vi "lectura comas2.vi"() -> ()   [LabVIEW 2021]
uses:
  <vilib>/Instr/_visa.llb/VISA Configure Serial Port (Instr).vi
panel:
  in  "PARO":bool
  in  "stop":bool
  out "BUFFER":string
  out "HUMEDAD":dbl(slide) scale=0.0..100.0
  out "TEMPERATURA":dbl(slide) scale=0.0..100.0
  in  "VISA resource name":refnum<visa-resource-name>
  in  "START":bool
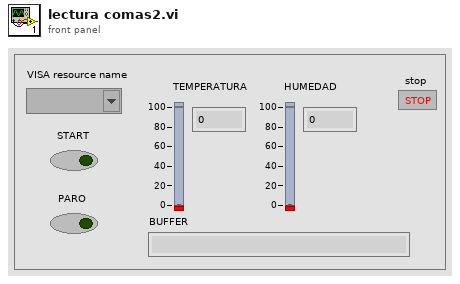
[diagram p1: front panel]
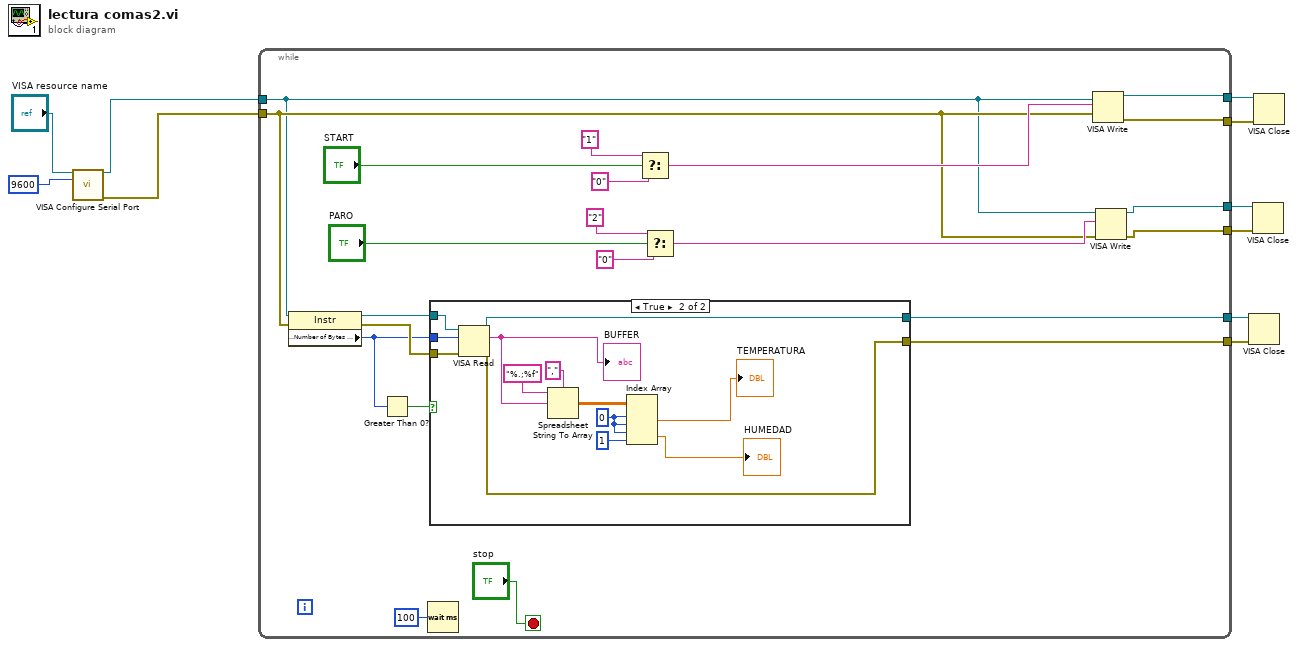
[diagram p0: block diagram]
diagram:
  n1 = call-poly "VISA Configure Serial Port"("VISA resource name"="VISA resource name", "baud rate (9600)"=u32 9600) -> ("VISA resource name out"=w10:refnum<visa-resource-name>, "error out"=w8:errorcluster)  [unwired: 12 in]
  n2 = while {
    tunnel: w10 -> [w13]
    tunnel: [w32] -> w9
    tunnel: w8 -> [w14]
    tunnel: [w31] -> w7
    tunnel: [w25] -> w4
    tunnel: [w24] -> w3
    tunnel: [w12] -> w2
    tunnel: [w11] -> w1
    stop <- "stop" stop-if-true
    n3 = property class="Instr"(reference=w13, error in=w14) -> (reference out=w21:refnum<visa-resource-name>, error out=w22:errorcluster, "Serial Settings:Number of Bytes at Serial Port"=w20:u32)
    n4 = Greater Than 0?(x=w20) -> (x > 0?=w19:bool)
    n5 = Wait (ms)(milliseconds to wait=u32 100) -> ()  [unwired: 1 out]
    n6 = case shown="True" w19 {
      tunnel: [w34 w39] -> w25
      tunnel: [w33 w38] -> w24
      tunnel: w22 -> [w33 w37]
      tunnel: w20 -> [_ w36]
      tunnel: w21 -> [w34 w35]
      frame False {
      }
      frame True {
        w44 = 0 ("index (row)")
        n7 = VISA Read(VISA resource name=w35, byte count=w36, error in (no error)=w37) -> (VISA resource name out=w39:refnum<visa-resource-name>, read buffer=w40:string, error out=w38:errorcluster)  [unwired: 1 out]
        "BUFFER" <- w40
        n8 = Spreadsheet String To Array(delimiter (Tab)=",", format string="%.;%f", spreadsheet string=w40) -> (array=w45:dbl[][])  [unwired: 1 in]
        n9 = Index Array(array=w45, index (row) #1=w44, index (col) #1=w44, index (row) #2=w44, index (col) #2=1 ("disabled index (col)")) -> (element #1=→"TEMPERATURA":dbl, element #2=→"HUMEDAD":dbl)
      }
    }
    n10 = Select(t="1", s="START", f="0") -> (s? t:f=w27:string)
    n11 = Select(t="2", s="PARO", f="0") -> (s? t:f=w15:string)
    n12 = VISA Write(VISA resource name=w13, write buffer=w27, error in (no error)=w14) -> (VISA resource name out=w32:refnum<visa-resource-name>, error out=w31:errorcluster)  [unwired: 1 out]
    n13 = VISA Write(VISA resource name=w13, write buffer=w15, error in (no error)=w14) -> (VISA resource name out=w12:refnum<visa-resource-name>, error out=w11:errorcluster)  [unwired: 1 out]
  }
  n14 = VISA Close(VISA resource name=w4, error in (no error)=w3) -> ()  [unwired: 1 out]
  n15 = VISA Close(VISA resource name=w2, error in (no error)=w1) -> ()  [unwired: 1 out]
  n16 = VISA Close(VISA resource name=w9, error in (no error)=w7) -> ()  [unwired: 1 out]
